vi "Get Decay Fit Parameters.vi"(7 "Laser Period":dbl, 10 "Decay Fit Output Options":T1, 11 "Decay Fit Parameters":dbl[](array[numeric])) -> (2 "Parameter Name Array":T3[](array[typedef]), 3 "Displayed Decay Fits Parameters":dbl[](array[numeric]))   [LabVIEW 2021, in "Fits.lvlib"]
doc: "Get Decay fit parameters from fir output."
uses:
  Fits.lvlib
  Decay Fit Parameters & Derived Quantities List.ctl
  AlliGator/AlliGator Decay Fit Output Options.ctl
  Decay Convolution/Decay Model.ctl
  Arrays/Arrays.lvlib
  AlliGator/AlliGator Decay Fit.lvlib
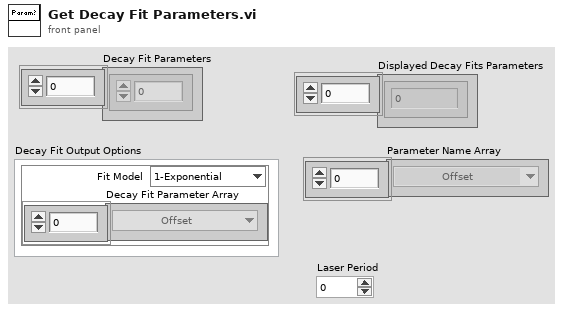
[diagram p1: front panel]
types:
  T1 = typedef "AlliGator Decay Analysis.lvlib/AlliGator Decay Fit.lvlib/AlliGator Decay Fit Output Options.ctl" = cluster{"Fit Model":T2, "Decay Fit Parameter Array":T3[]}
  T2 = typedef "Fits.lvlib/Decay Model.ctl" = enum16{"1-Exponential", "2-Exponentials"}
  T3 = typedef "Fits.lvlib/Decay Fit Parameters & Derived Quantities List.ctl" = enum16{"Offset", "Baseline", "A_1", "tau_1", "A_2", "tau_2", "<tau>_a", "f1_a", "f2_a", "<tau>_i", "f1_i", "f2_i", "-", "R^2", "Chi^2"}
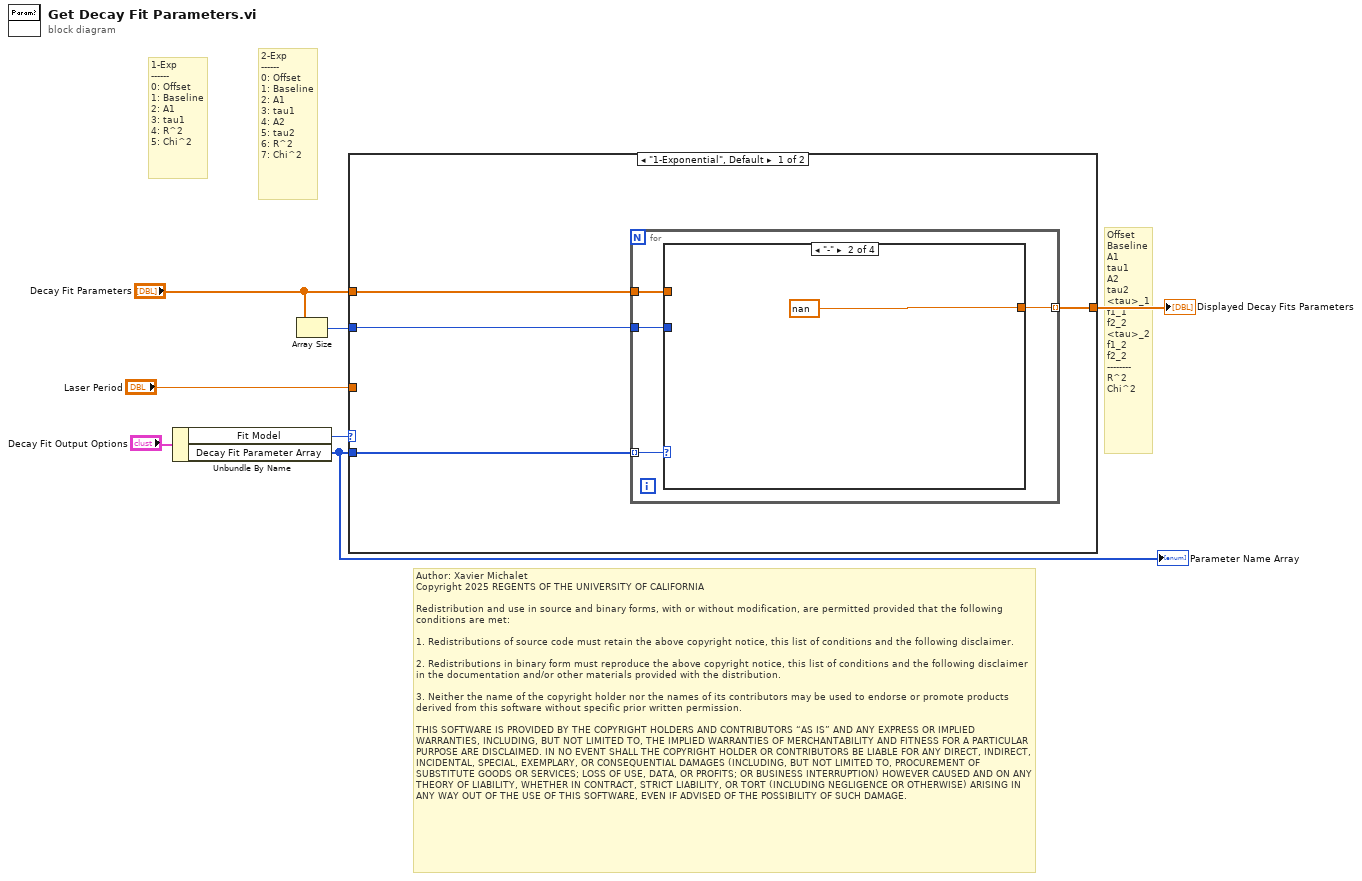
[diagram p0: block diagram]
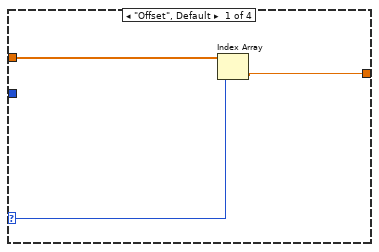
[diagram p2: hidden frame]
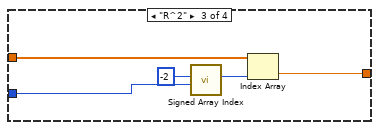
[diagram p3: hidden frame]
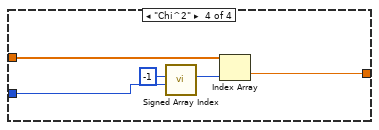
[diagram p4: hidden frame]
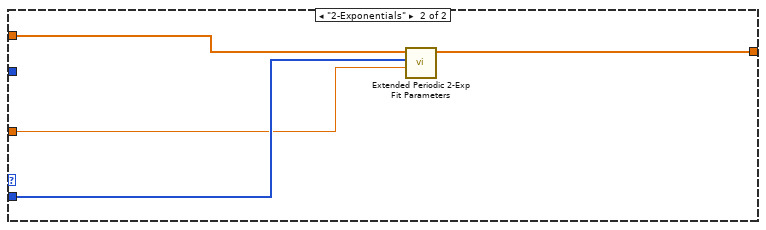
[diagram p5: hidden frame]
diagram:
  # "Author: Xavier Michalet\nCopyright 2025 REGENTS OF THE UNIVERSITY OF CALIFORNIA\n\nRedistribution and use in source and binary forms, with or without modification, are permitted provided that the following conditions are met:\n\n1. Redistributions of source code must retain the above copyright notice, this list of conditions and the following disclaimer.\n\n2. Redistributions in binary form must reproduce the above copyright notice, this list of conditions and the following disclaimer in the documentation and/or other materials provided with the distribution.\n\n3. Neither the name of the copyright holder nor the names of its contributors may be used to endorse or promote products derived from this software without specific prior written permission.\n\nTHIS SOFTWARE IS PROVIDED BY THE COPYRIGHT HOLDERS AND CONTRIBUTORS “AS IS” AND ANY EXPRESS OR IMPLIED WARRANTIES, INCLUDING, BUT NOT LIMITED TO, THE IMPLIED WARRANTIES OF MERCHANTABILITY AND FITNESS FOR A PARTICULAR PURPOSE ARE DISCLAIMED. IN NO EVENT SHALL THE COPYRIGHT HOLDER OR CONTRIBUTORS BE LIABLE FOR ANY DIRECT, INDIRECT, INCIDENTAL, SPECIAL, EXEMPLARY, OR CONSEQUENTIAL DAMAGES (INCLUDING, BUT NOT LIMITED TO, PROCUREMENT OF SUBSTITUTE GOODS OR SERVICES; LOSS OF USE, DATA, OR PROFITS; OR BUSINESS INTERRUPTION) HOWEVER CAUSED AND ON ANY THEORY OF LIABILITY, WHETHER IN CONTRACT, STRICT LIABILITY, OR TORT (INCLUDING NEGLIGENCE OR OTHERWISE) ARISING IN ANY WAY OUT OF THE USE OF THIS SOFTWARE, EVEN IF ADVISED OF THE POSSIBILITY OF SUCH DAMAGE."
  # "1-Exp\n------\n0: Offset\n1: Baseline\n2: A1\n3: tau1\n4: R^2\n5: Chi^2"
  # "2-Exp\n------\n0: Offset\n1: Baseline\n2: A1\n3: tau1\n4: A2\n5: tau2\n6: R^2\n7: Chi^2"
  # "Offset\nBaseline\nA1\ntau1\nA2\ntau2\n<tau>_1\nf1_1\nf2_2\n<tau>_2\nf1_2\nf2_2\n--------\nR^2\nChi^2"
  n1 = Unbundle By Name("Decay Fit Output Options") -> ("Fit Model"=w4:T2, "Decay Fit Parameter Array"=w2:T3[])
  "Parameter Name Array" <- w2
  n2 = Array Size(array="Decay Fit Parameters") -> (size(s)=w5:i32)
  n3 = case shown="\"1-Exponential\", Default" w4 {
    tunnel: [w10 w33] -> w7
    tunnel: "Decay Fit Parameters" -> [w11 w32]
    tunnel: w2 -> [w8 w31]
    tunnel: w5 -> [w9 _]
    tunnel: "Laser Period" -> [_ w30]
    frame "1-Exponential", Default {
      n4 = for {
        tunnel: w8 -> [w15] mode=indexing
        tunnel: w11 -> [w14]
        tunnel: [w13] -> w10 mode=indexing
        tunnel: w9 -> [w12]
        n5 = case shown="\"-\"" w15 {
          selector: w15 -> [w17 _ _ _]
          tunnel: w14 -> [w18 _ w23 w27]
          tunnel: [w16 nan ("Numeric") w21 w25] -> w13
          tunnel: w12 -> [_ _ w24 w26]
          frame "Offset", Default {
            n6 = Index Array(array=w18, index=w17) -> (element=w16:dbl)
          }
          frame "-" {
          }
          frame "R^2" {
            n7 = call "Signed Array Index.vi"("Array Size"=w24, "Array Index in"=-2) -> ("Array Index out"=w22:i32)  [unwired: 9 in]
            n8 = Index Array(array=w23, index=w22) -> (element=w21:dbl)
          }
          frame "Chi^2" {
            n9 = call "Signed Array Index.vi"("Array Size"=w26, "Array Index in"=-1) -> ("Array Index out"=w29:i32)  [unwired: 9 in]
            n10 = Index Array(array=w27, index=w29) -> (element=w25:dbl)
          }
        }
      }
    }
    frame "2-Exponentials" {
      n11 = call "Extended Periodic 2-Exp Fit Parameters.vi"("Laser Period"=w30, "Selected Decay Fit Parameter Array"=w31, "Decay Fit Parameters"=w32) -> ("Extended Decay Fit Parameters"=w33:dbl[])  [unwired: 7 in, 1 out]
    }
  }
  "Displayed Decay Fits Parameters" <- w7
